vi "Status Write stop_com.vi"(8 "error in (no error)":errorcluster, 9 "Stop":bool, 11 "Status References":T1[](array[typedef])) -> (0 "error out":errorcluster, 3 "Status References out":T1[](array[typedef]))   [LabVIEW 2019, in "Status.lvlib"]
uses:
  Status.lvlib
  Ctl/control.ctl
  Ctl/State.ctl
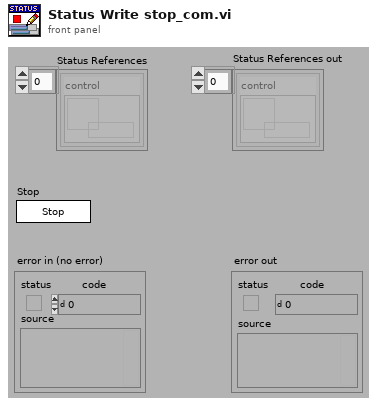
[diagram p1: front panel]
types:
  T1 = typedef "Status.lvlib/control.ctl" = cluster{"control":refnum<data-value>}
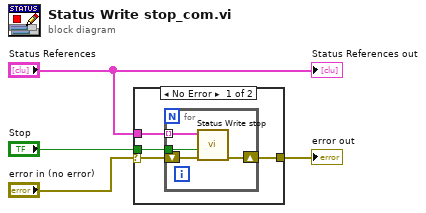
[diagram p0: block diagram]
diagram:
  n1 = case shown="No Error" "error in (no error)" {
    selector: "error in (no error)" -> [w8 w13]
    tunnel: [w7 w13] -> w1
    tunnel: "Status References" -> [w6 _]
    tunnel: "Stop" -> [w5 _]
    frame No Error {
      n2 = for {
        shift-right: [w11] -> w7
        shift-left: w8 -> [w12]
        tunnel: w6 -> [w10] mode=indexing
        tunnel: w5 -> [w9]
        n3 = call "Status Write stop.vi"("error in (no error)"=w12, "Stop"=w9, "Status Reference"=w10) -> ("error out"=w11:errorcluster)  [unwired: 7 in, 1 out]
      }
    }
    frame Error {
    }
  }
  "error out" <- w1
  "Status References out" <- "Status References"
